vi "IOExtract.vi"(0 "Instrument(Number):":i32 min=0 max=9999, 1 "Instrument(String)":string) -> (2 "InterfaceCode:\n0: GPIB\n1: ISOBUS":i32, 3 "FunctionCode:":i32, 4 "Address":i32)   [LabVIEW 2012]
doc: "Interface code:\n 0: GIPB\n 1: ISOBUS\nFunction code:\nAddress:"
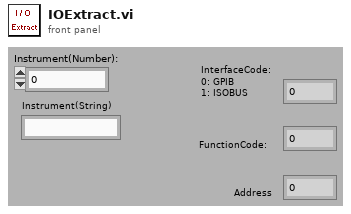
[diagram p1: front panel]
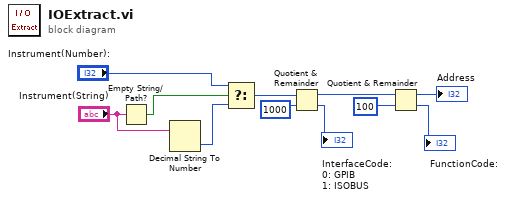
[diagram p0: block diagram]
diagram:
  n1 = Empty String/Path?(string/path="Instrument(String)") -> (empty?=w11:bool)
  n2 = Decimal String To Number(string="Instrument(String)") -> (number=w9:i32)  [unwired: 2 in, 1 out]
  n3 = Select(t="Instrument(Number):", s=w11, f=w9) -> (s? t:f=w7:i32)
  n4 = Quotient & Remainder(x=w7, y=1000) -> (x-y*floor(x/y)=w3:i32, floor(x/y)=→"InterfaceCode:\n0: GPIB\n1: ISOBUS":i32)
  n5 = Quotient & Remainder(x=w3, y=100) -> (x-y*floor(x/y)=→"Address":i32, floor(x/y)=→"FunctionCode:":i32)
